vi "Counters.vi"(0 "DigitalInputs":bool[](array[boolean])=[FALSE, FALSE, FALSE, FALSE, FALSE, FALSE, FALSE, FALSE, FALSE, FALSE, FALSE, FALSE, FALSE, FALSE, FALSE, FALSE, FALSE, FALSE, FALSE, FALSE, FALSE, FALSE, FALSE, FALSE, FALSE, FALSE, FALSE, FALSE, FALSE, FALSE, FALSE, FALSE], 1 "AnalogTriggers":T3[](array[typedef])=[{"InHysteresis"=FALSE, "OverLimit"=FALSE, "Rising"=FALSE, "Falling"=FALSE}, {"InHysteresis"=FALSE, "OverLimit"=FALSE, "Rising"=FALSE, "Falling"=FALSE}, {"InHysteresis"=FALSE, "OverLimit"=FALSE, "Rising"=FALSE, "Falling"=FALSE}, {"InHysteresis"=FALSE, "OverLimit"=FALSE, "Rising"=FALSE, "Falling"=FALSE}, {"InHysteresis"=FALSE, "OverLimit"=FALSE, "Rising"=FALSE, "Falling"=FALSE}, {"InHysteresis"=FALSE, "OverLimit"=FALSE, "Rising"=FALSE, "Falling"=FALSE}, {"InHysteresis"=FALSE, "OverLimit"=FALSE, "Rising"=FALSE, "Falling"=FALSE}, {"InHysteresis"=FALSE, "OverLimit"=FALSE, "Rising"=FALSE, "Falling"=FALSE}], 2 "Counter_TimerConfigs":T7, 3 "Configs":T9, 4 "Resets":T4) -> (5 "Counter_Outputs":T1, 6 "Counter_TimerOutputs":T5)   [LabVIEW 2019]
uses:
  Controls/Counter_Configs.ctl
  Controls/Counter_Config.ctl
  Helpers/Source.ctl
  Controls/Counter_TimerConfigs.ctl
  Controls/TimerConfig.ctl
  Controls/Counter_TimerOutputs.ctl
  Helpers/TimerOutput.ctl
  Controls/Counter_Resets.ctl
  Helpers/AnalogTriggerOutput.ctl
  Controls/Counter_Outputs.ctl
  Controls/Counter_Output.ctl
  <vilib>/rvi/Emulation/niFpgaSctlEmulationGetInTimedLoop.vi
  <vilib>/rvi/Emulation/niFpgaProcessEmulError.vi
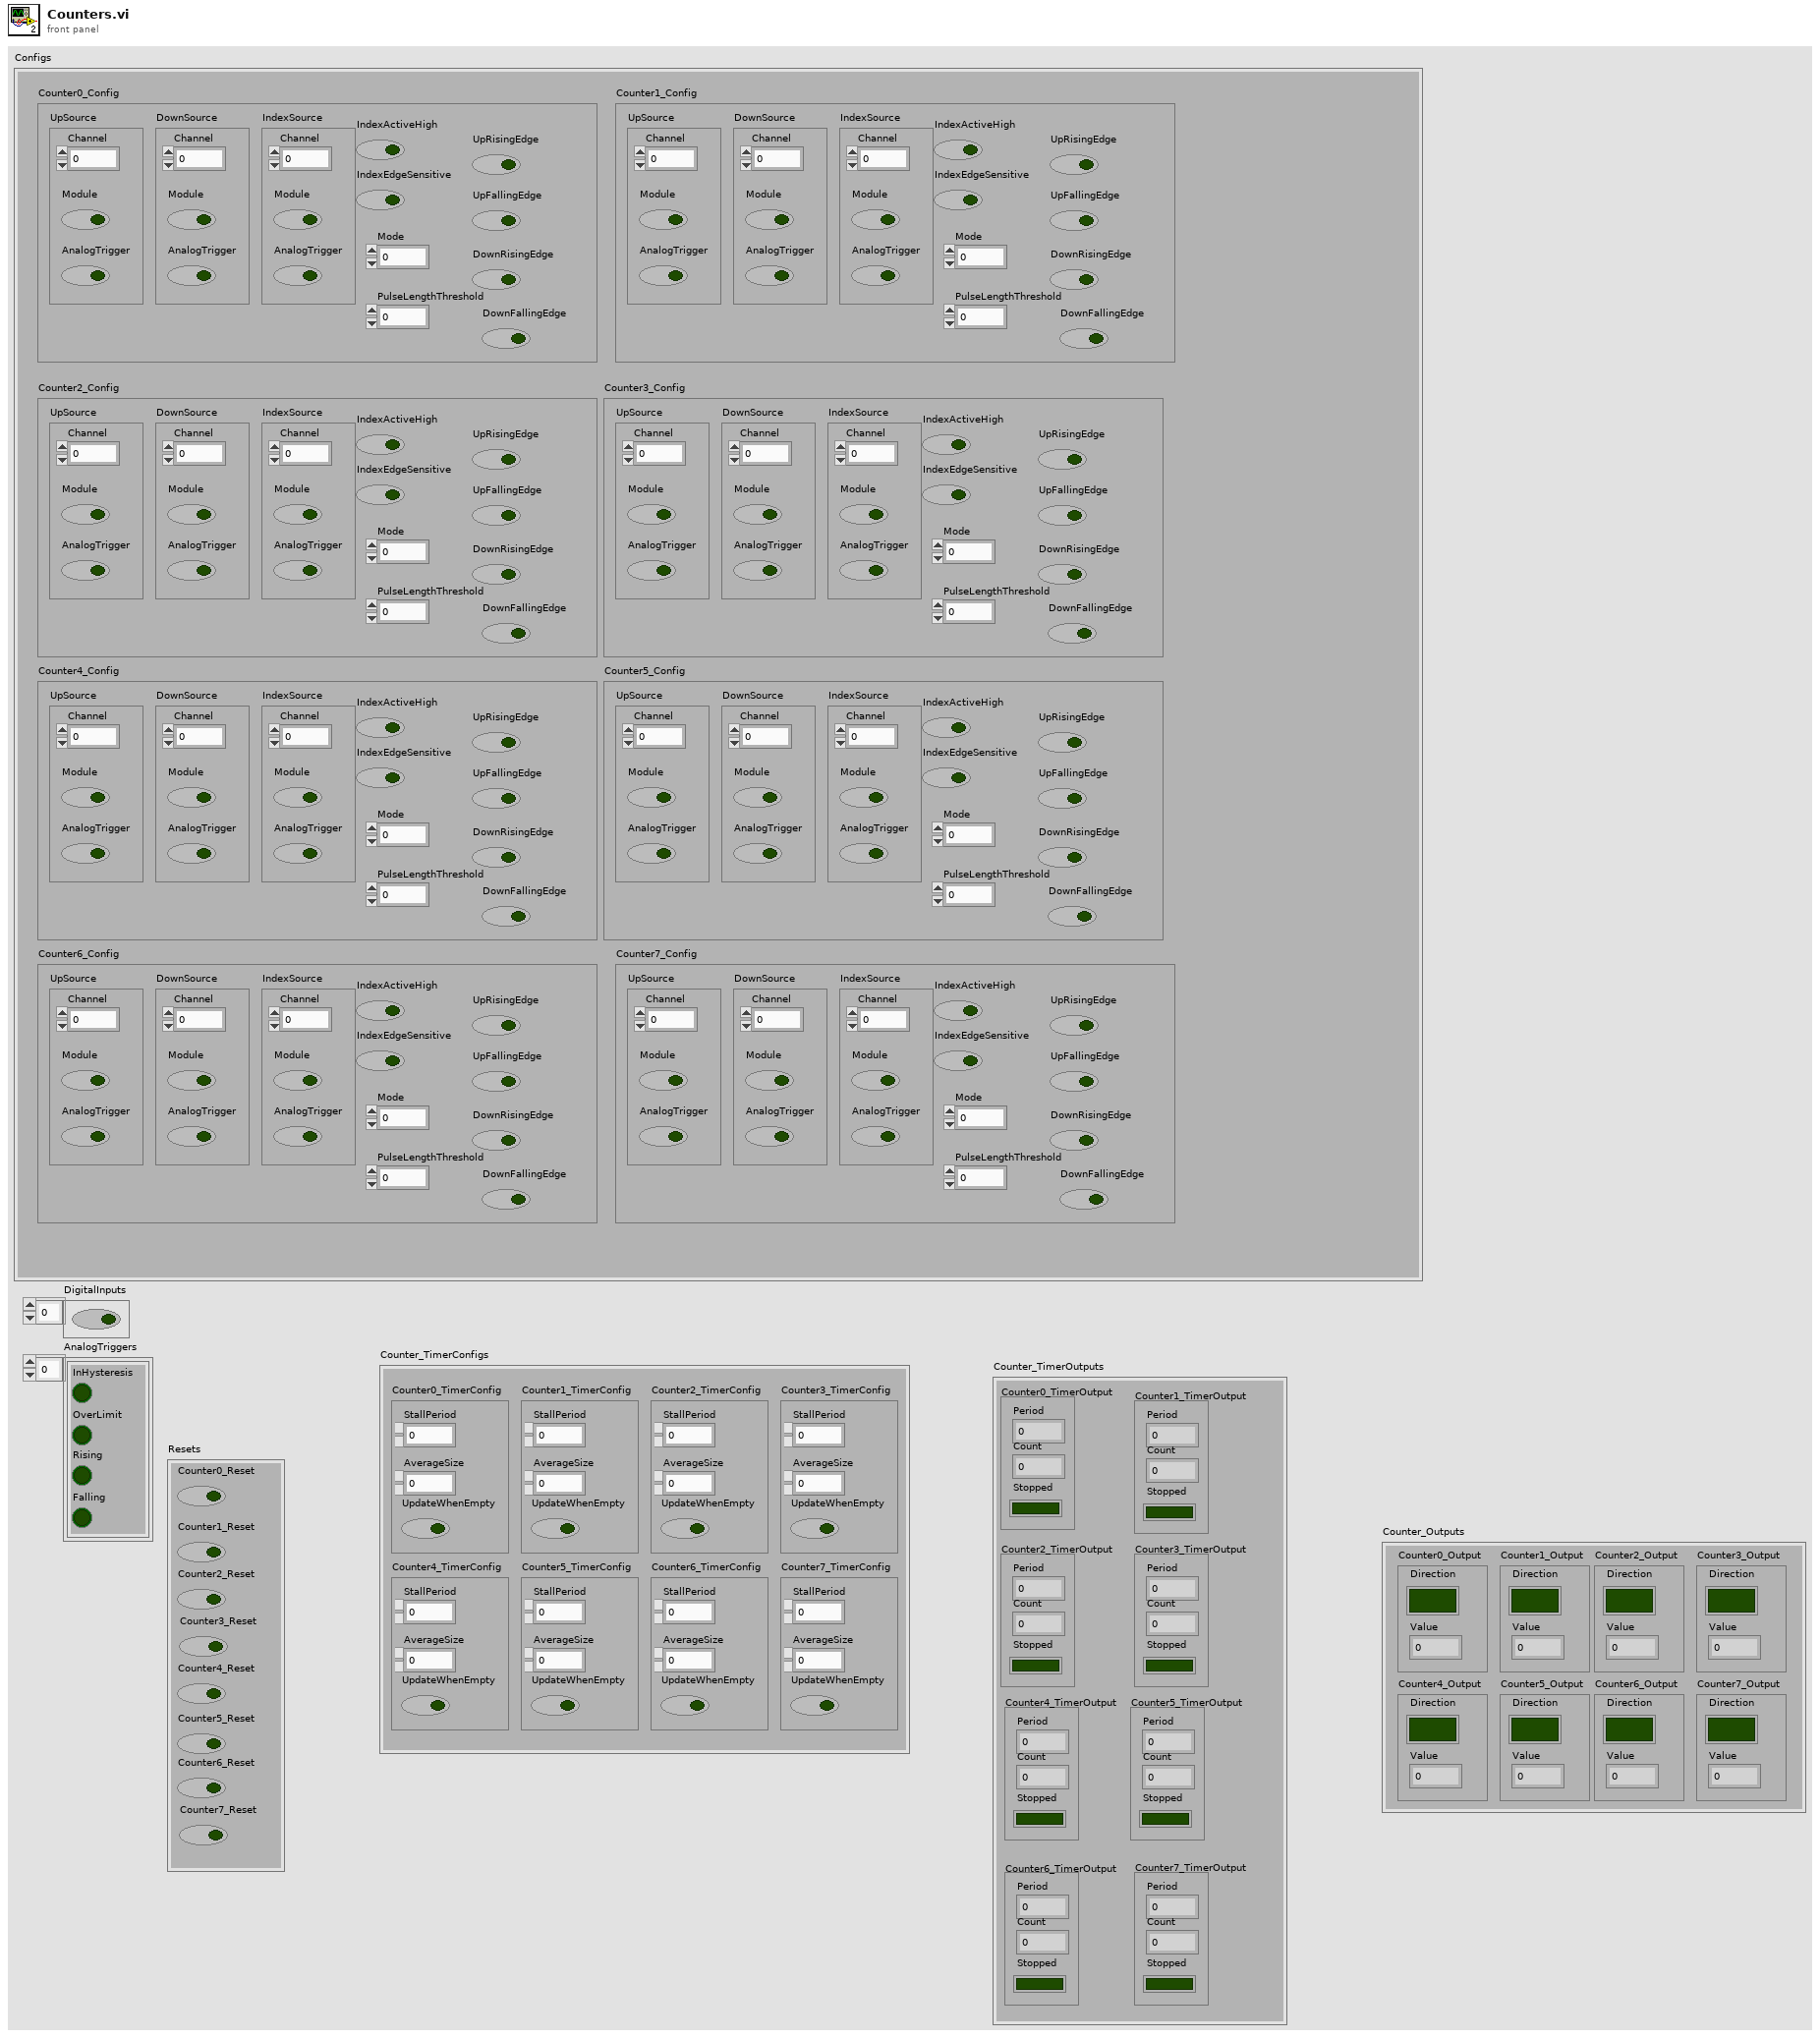
[diagram p1: front panel]
types:
  T1 = typedef "Counter_Outputs.ctl" = cluster{"Counter0_Output":T2, "Counter1_Output":T2, "Counter2_Output":T2, "Counter3_Output":T2, "Counter4_Output":T2, "Counter5_Output":T2, "Counter6_Output":T2, "Counter7_Output":T2}
  T2 = typedef "Counter_Output.ctl" = cluster{"Direction":bool, "Value":fxp<+/-,31,31>}
  T3 = typedef "AnalogTriggerOutput.ctl" = cluster{"InHysteresis":bool, "OverLimit":bool, "Rising":bool, "Falling":bool}
  T4 = typedef "Counter_Resets.ctl" = cluster{"Counter0_Reset":bool, "Counter1_Reset":bool, "Counter2_Reset":bool, "Counter3_Reset":bool, "Counter4_Reset":bool, "Counter5_Reset":bool, "Counter6_Reset":bool, "Counter7_Reset":bool}
  T5 = typedef "Counter_TimerOutputs.ctl" = cluster{"Counter0_TimerOutput":T6, "Counter1_TimerOutput":T6, "Counter2_TimerOutput":T6, "Counter3_TimerOutput":T6, "Counter4_TimerOutput":T6, "Counter5_TimerOutput":T6, "Counter6_TimerOutput":T6, "Counter7_TimerOutput":T6}
  T6 = typedef "TimerOutput.ctl" = cluster{"Period":fxp<+,24,25>, "Count":i16, "Stopped":bool}
  T7 = typedef "Counter_TimerConfigs.ctl" = cluster{"Counter0_TimerConfig":T8, "Counter1_TimerConfig":T8, "Counter2_TimerConfig":T8, "Counter3_TimerConfig":T8, "Counter4_TimerConfig":T8, "Counter5_TimerConfig":T8, "Counter6_TimerConfig":T8, "Counter7_TimerConfig":T8}
  T8 = typedef "TimerConfig.ctl" = cluster{"StallPeriod":fxp<+,24,24>, "AverageSize":fxp<+,7,7>, "UpdateWhenEmpty":bool}
  T9 = typedef "Counter_Configs.ctl" = cluster{"Counter0_Config":T10, "Counter1_Config":T10, "Counter2_Config":T10, "Counter3_Config":T10, "Counter4_Config":T10, "Counter5_Config":T10, "Counter6_Config":T10, "Counter7_Config":T10}
  T10 = typedef "Counter_Config.ctl" = cluster{"UpSource":T11, "DownSource":T11, "IndexSource":T11, "IndexActiveHigh":bool, "IndexEdgeSensitive":bool, "UpRisingEdge":bool, "UpFallingEdge":bool, "DownRisingEdge":bool, "DownFallingEdge":bool, "Mode":fxp<+,2,2>, "PulseLengthThreshold":fxp<+,6,14>}
  T11 = typedef "Source.ctl" = cluster{"Channel":fxp<+,4,4>, "Module":bool, "AnalogTrigger":bool}
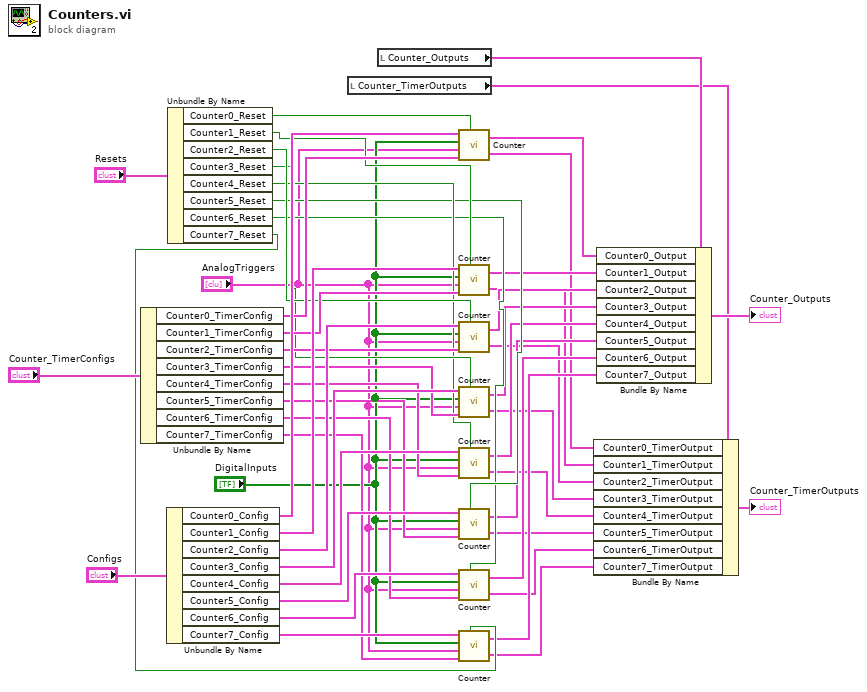
[diagram p0: block diagram]
diagram:
  n1 = Unbundle By Name("Counter_TimerConfigs") -> ("Counter0_TimerConfig"=w39:T8, "Counter1_TimerConfig"=w38:T8, "Counter2_TimerConfig"=w37:T8, "Counter3_TimerConfig"=w36:T8, "Counter4_TimerConfig"=w35:T8, "Counter5_TimerConfig"=w34:T8, "Counter6_TimerConfig"=w33:T8, "Counter7_TimerConfig"=w32:T8)
  n2 = Unbundle By Name("Configs") -> ("Counter0_Config"=w48:T10, "Counter1_Config"=w47:T10, "Counter2_Config"=w46:T10, "Counter3_Config"=w45:T10, "Counter4_Config"=w44:T10, "Counter5_Config"=w43:T10, "Counter6_Config"=w42:T10, "Counter7_Config"=w41:T10)
  n3 = Unbundle By Name("Resets") -> ("Counter0_Reset"=w30:bool, "Counter1_Reset"=w29:bool, "Counter2_Reset"=w28:bool, "Counter3_Reset"=w27:bool, "Counter4_Reset"=w26:bool, "Counter5_Reset"=w25:bool, "Counter6_Reset"=w24:bool, "Counter7_Reset"=w23:bool)
  n4 = local read "Counter_TimerOutputs"() -> (w9:T5)
  n5 = local read "Counter_Outputs"() -> (w20:T1)
  n6 = call "Counter.vi"("Reset"=w30, "TimerConfig"=w39, "AnalogTriggers"="AnalogTriggers", "DigitalInputs"="DigitalInputs", "Config"=w48) -> ("TimerOutput"=w8:T6, "Output"=w19:T2)  [unwired: 1 in]
  n7 = call "Counter.vi"("Reset"=w29, "TimerConfig"=w38, "AnalogTriggers"="AnalogTriggers", "DigitalInputs"="DigitalInputs", "Config"=w47) -> ("TimerOutput"=w7:T6, "Output"=w18:T2)  [unwired: 1 in]
  n8 = call "Counter.vi"("Reset"=w28, "TimerConfig"=w37, "AnalogTriggers"="AnalogTriggers", "DigitalInputs"="DigitalInputs", "Config"=w46) -> ("TimerOutput"=w6:T6, "Output"=w17:T2)  [unwired: 1 in]
  n9 = call "Counter.vi"("Reset"=w27, "TimerConfig"=w36, "AnalogTriggers"="AnalogTriggers", "DigitalInputs"="DigitalInputs", "Config"=w45) -> ("TimerOutput"=w5:T6, "Output"=w16:T2)  [unwired: 1 in]
  n10 = call "Counter.vi"("Reset"=w26, "TimerConfig"=w35, "AnalogTriggers"="AnalogTriggers", "DigitalInputs"="DigitalInputs", "Config"=w44) -> ("TimerOutput"=w4:T6, "Output"=w15:T2)  [unwired: 1 in]
  n11 = call "Counter.vi"("Reset"=w25, "TimerConfig"=w34, "AnalogTriggers"="AnalogTriggers", "DigitalInputs"="DigitalInputs", "Config"=w43) -> ("TimerOutput"=w3:T6, "Output"=w14:T2)  [unwired: 1 in]
  n12 = call "Counter.vi"("Reset"=w24, "TimerConfig"=w33, "AnalogTriggers"="AnalogTriggers", "DigitalInputs"="DigitalInputs", "Config"=w42) -> ("TimerOutput"=w2:T6, "Output"=w13:T2)  [unwired: 1 in]
  n13 = call "Counter.vi"("Reset"=w23, "TimerConfig"=w32, "AnalogTriggers"="AnalogTriggers", "DigitalInputs"="DigitalInputs", "Config"=w41) -> ("TimerOutput"=w1:T6, "Output"=w12:T2)  [unwired: 1 in]
  n14 = Bundle By Name(cluster=w9, "Counter0_TimerOutput"=w8, "Counter1_TimerOutput"=w7, "Counter2_TimerOutput"=w6, "Counter3_TimerOutput"=w5, "Counter4_TimerOutput"=w4, "Counter5_TimerOutput"=w3, "Counter6_TimerOutput"=w2, "Counter7_TimerOutput"=w1) -> (→"Counter_TimerOutputs":T5)
  n15 = Bundle By Name(cluster=w20, "Counter0_Output"=w19, "Counter1_Output"=w18, "Counter2_Output"=w17, "Counter3_Output"=w16, "Counter4_Output"=w15, "Counter5_Output"=w14, "Counter6_Output"=w13, "Counter7_Output"=w12) -> (→"Counter_Outputs":T1)
